vi "Data Acquisition.vi"() -> ()   [LabVIEW 2009]
panel:
  in  "Thresholding Cluster":T1={"F_DEx"=35, "F_AA"=35, " No of Bins"=100}
  out "output cluster":T2
  out "Histogram":dbl[][](graph) caption="Intensity Graph"
  in  "Current Configuration":i32
  in  "Configurations":T3(array[cluster])=[{"Configuration File Path"=path "", "Current Configuration"=TRUE}]
  in  "Time Bin (ms)":dbl=1.0 format="%.2f"
  out "APD Chart":i32[][](graph)=[[10, 21, 11, 14]]
  out "Current File Path":path
  out "Files Left To Acquire":i32
  in  "Data File I/O Information":T4={"Name of Configuration"="", "Path"=path "D:/User/Geraint/10_03_04", "File Name"="T1B18_GCW180_RAlt30um_20um_25mins_20pm_OpenAperture", "Files To Acquire"=1, "Current File Number"=3, "Time Limit"=1500.0, "Save Data"=TRUE, "Additional Comments"=""}
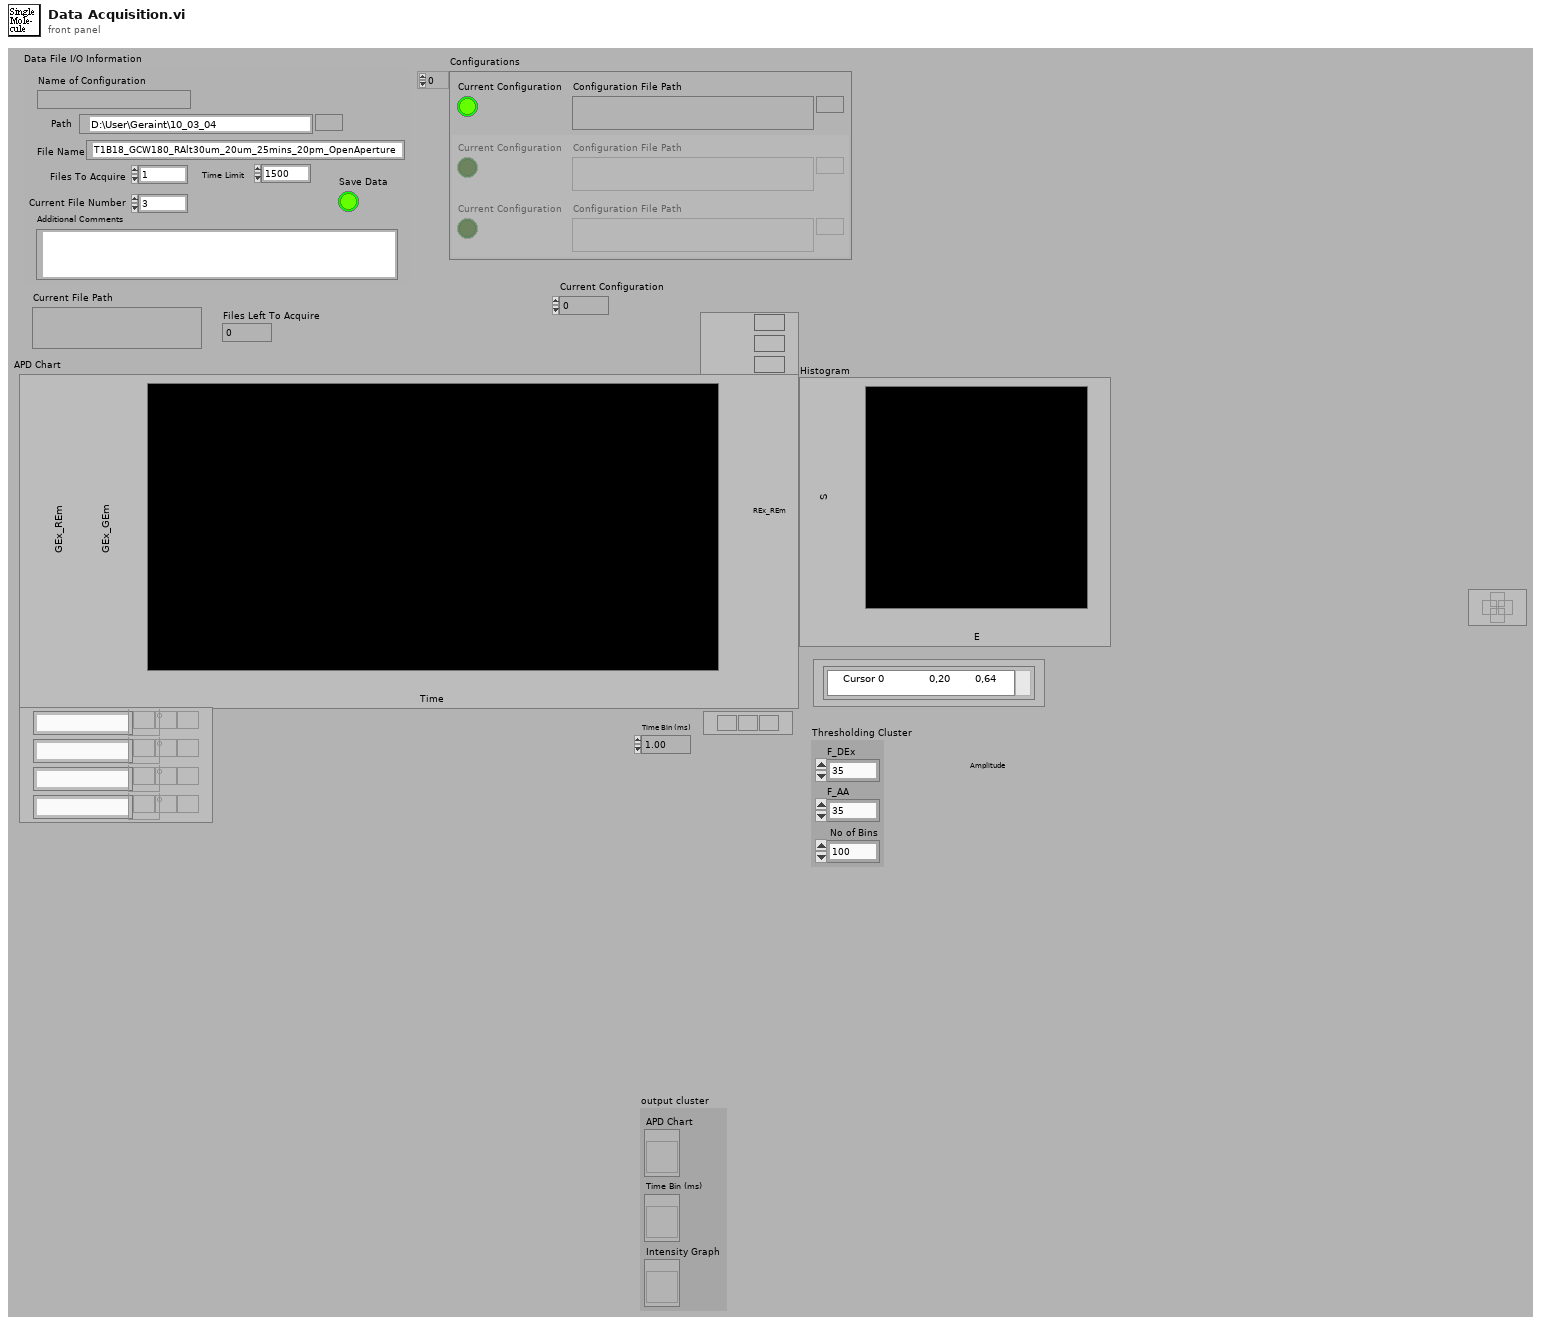
[diagram p1: front panel]
types:
  T1 = cluster{"F_DEx":i32, "F_AA":i32, " No of Bins":i32}
  T2 = cluster{"APD Chart":refnum<vi>, "Time Bin (ms)":refnum<vi>, "Intensity Graph":refnum<vi>}
  T3 = cluster{"Configuration File Path":path, "Current Configuration":bool}[]
  T4 = cluster{"Name of Configuration":string, "Path":path, "File Name":string, "Files To Acquire":i32, "Current File Number":i32, "Time Limit":dbl, "Save Data":bool, "Additional Comments":string}
  T5 = cluster{"Configuration File Path":path, "Current Configuration":bool}
  T6 = cluster{"APD Chart":refnum<vi>, "Time Bin (ms)":refnum<vi>, "Histogram":refnum<vi>}
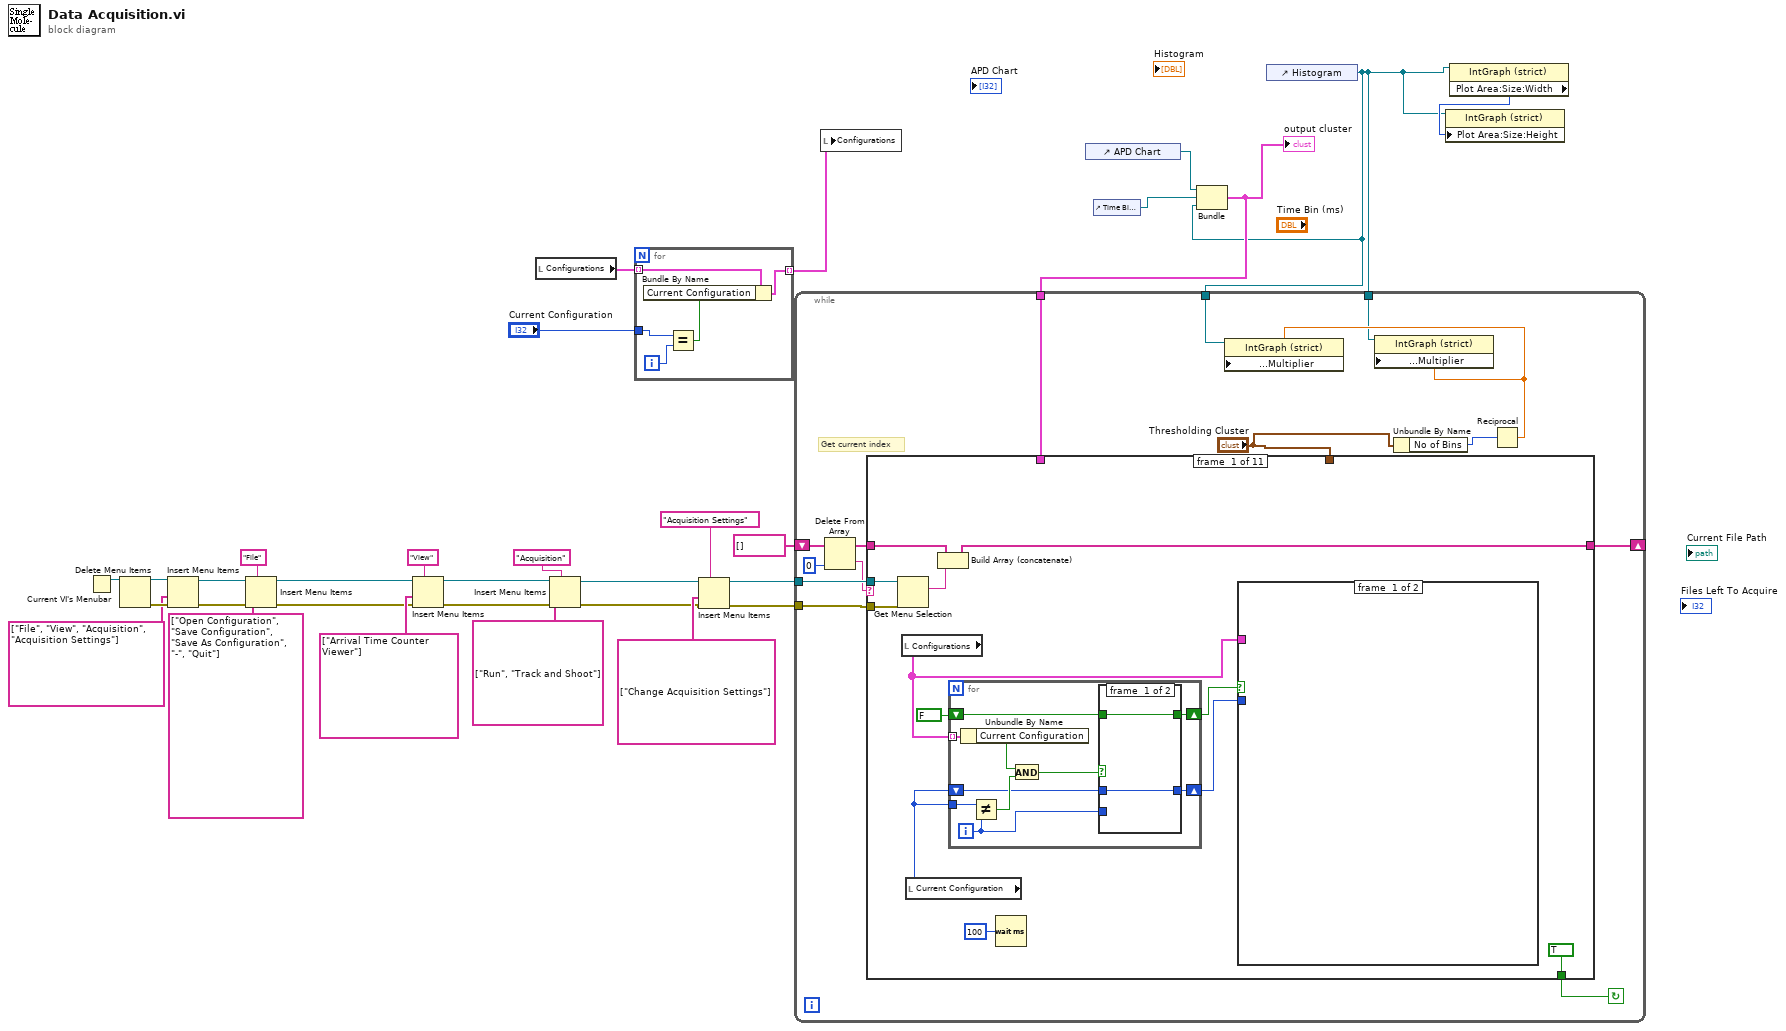
[diagram p0: block diagram]
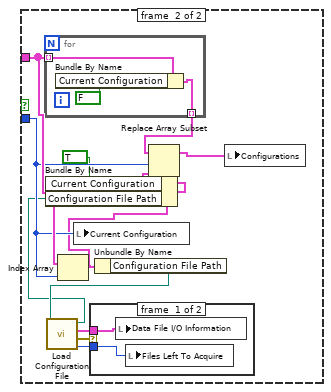
[diagram p2: hidden frame]
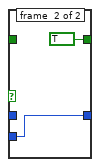
[diagram p4: hidden frame]
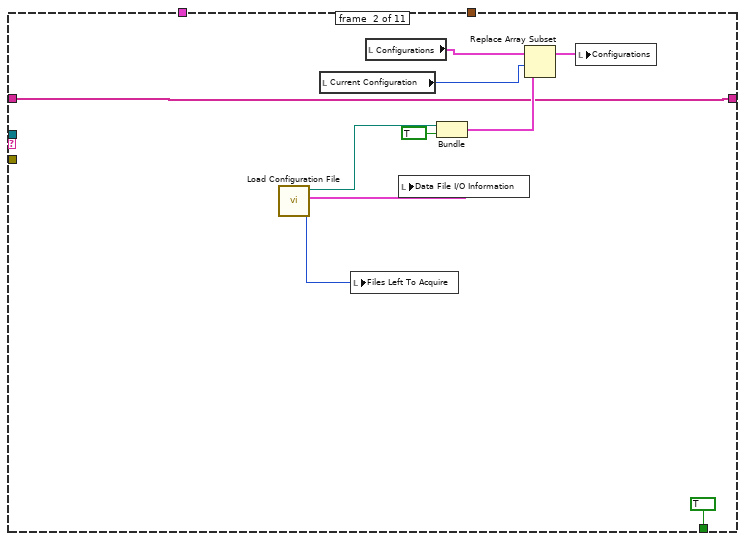
[diagram p5: hidden frame]
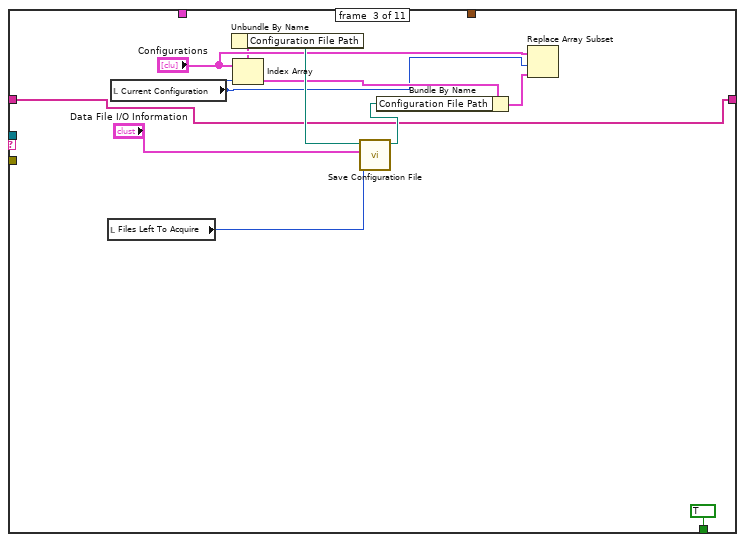
[diagram p6: hidden frame]
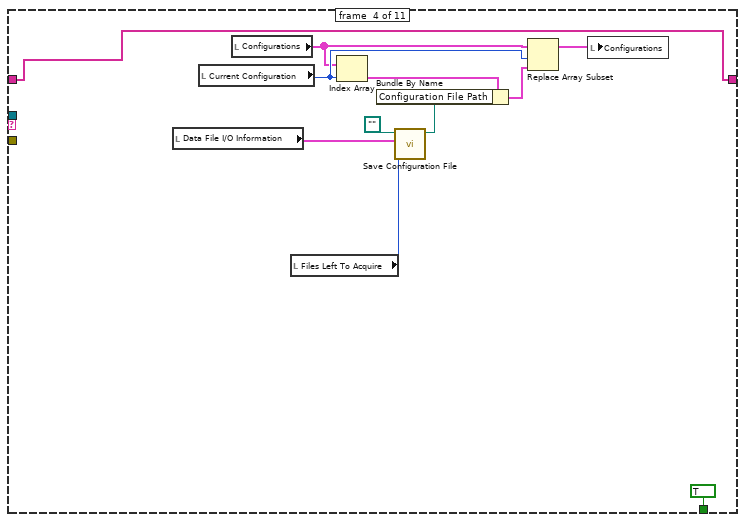
[diagram p7: hidden frame]
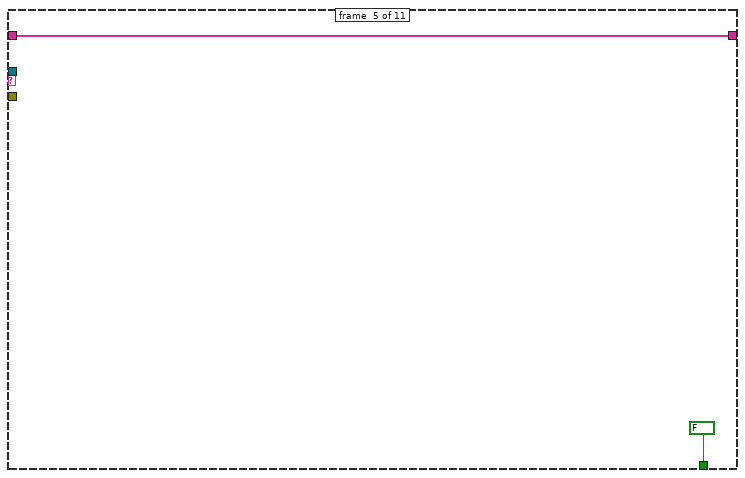
[diagram p8: hidden frame]
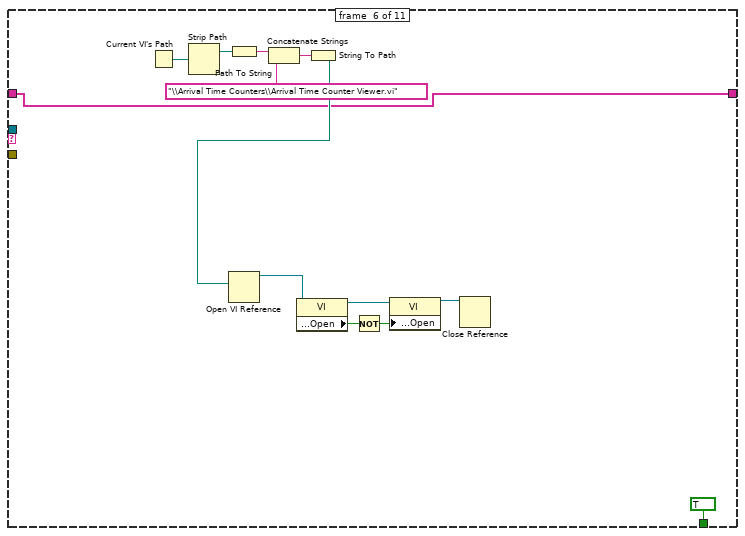
[diagram p9: hidden frame]
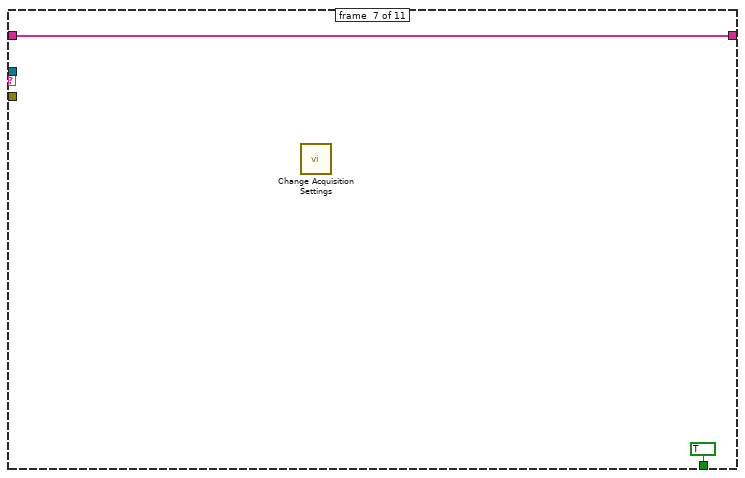
[diagram p10: hidden frame]
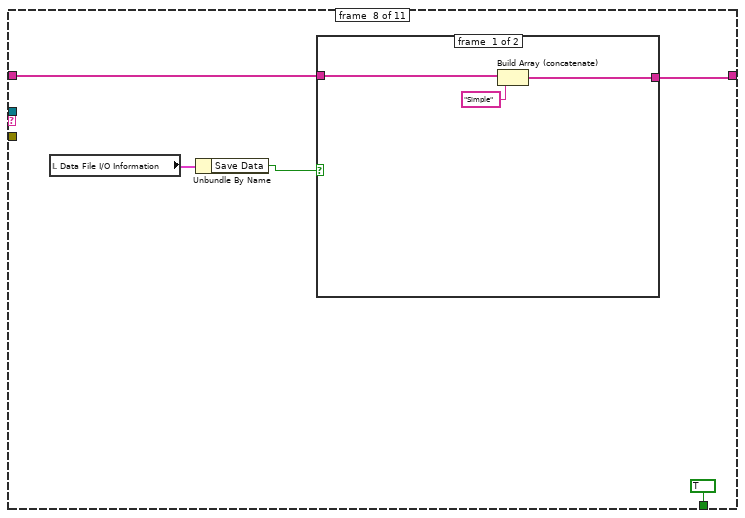
[diagram p11: hidden frame]
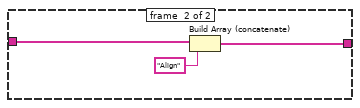
[diagram p12: hidden frame]
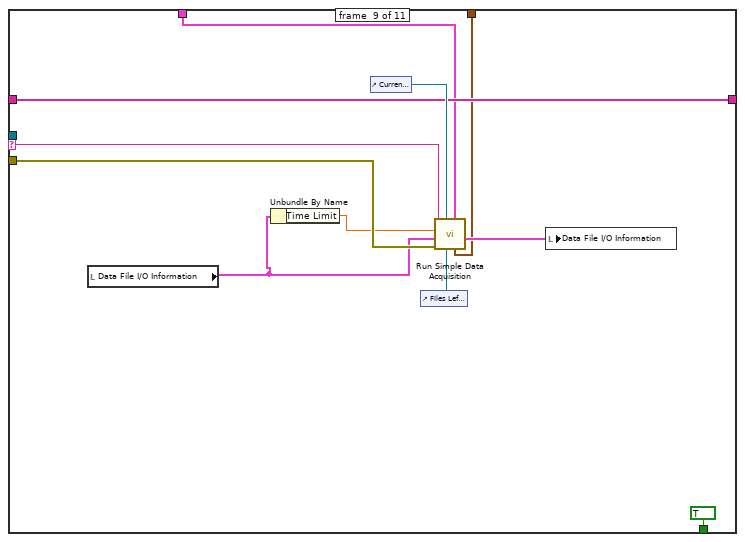
[diagram p13: hidden frame]
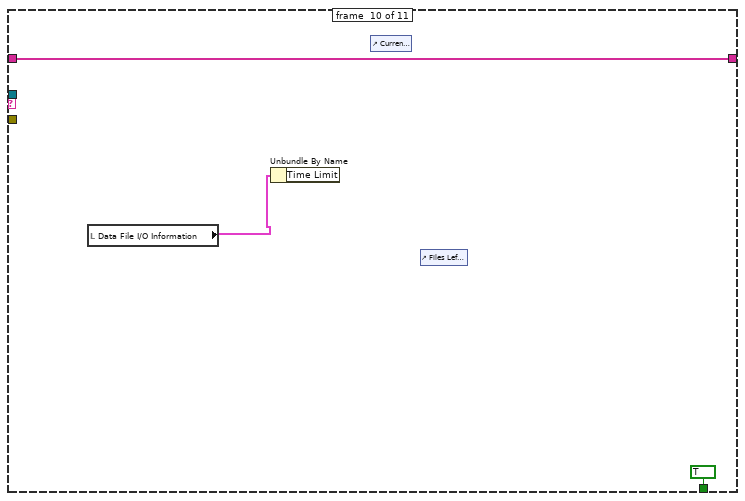
[diagram p14: hidden frame]
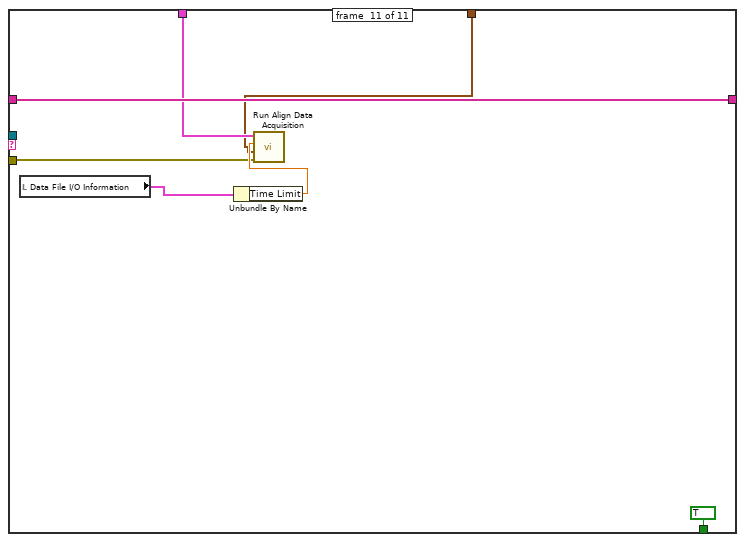
[diagram p15: hidden frame]
diagram:
  n1 = Current VI's Menubar() -> (w31:refnum<k9>)
  n2 = Delete Menu Items(9:w31) -> (0:w26:errorcluster, 3:w27:refnum<k9>)  [unwired: 3 in]
  n3 = Insert Menu Items(6:w26, 7:string[] ["File", "View", "Acquisition", "Acquisition Settings"] ("item tags"), 9:w27) -> (0:w25:errorcluster, 3:w28:refnum<k9>)  [unwired: 3 in, 1 out]
  n4 = Insert Menu Items(5:"File" ("menu tag"), 6:w25, 7:string[] ["Open Configuration", "Save Configuration", "Save As Configuration", "-", "Quit"] ("item tags"), 9:w28) -> (0:w16:errorcluster, 3:w17:refnum<k9>)  [unwired: 2 in, 1 out]
  n5 = Insert Menu Items(5:"View" ("menu tag"), 6:w16, 7:string[] ["Arrival Time Counter Viewer"] ("item tags"), 9:w17) -> (0:w15:errorcluster, 3:w14:refnum<k9>)  [unwired: 2 in, 1 out]
  n6 = local read "Configurations"() -> (w8:T3)
  n7 = Insert Menu Items(5:"Acquisition" ("menu tag"), 6:w15, 7:string[] ["Run", "Track and Shoot"] ("item tags"), 9:w14) -> (0:w12:errorcluster, 3:w13:refnum<k9>)  [unwired: 2 in, 1 out]
  n8 = for {
    tunnel: w8 -> [w36] mode=indexing
    tunnel: "Current Configuration" -> [w35]
    tunnel: [w32] -> w6 mode=indexing
    i -> [w34]
    n9 = Equal?(x=w35, y=w34) -> (x = y?=w33:bool)
    n10 = Bundle By Name(cluster=w36, "Current Configuration"=w33) -> (w32:T5)
  }
  n11 = Insert Menu Items(5:"Acquisition Settings" ("menu tag"), 6:w12, 7:string[] ["Change Acquisition Settings"] ("item tags"), 9:w13) -> (0:w10:errorcluster, 3:w11:refnum<k9>)  [unwired: 2 in, 1 out]
  n12 = local write "Configurations"(w6) -> ()
  n13 = control-ref of="APD Chart"() -> (w3:refnum<vi>)
  n14 = control-ref of="Time Bin (ms)"() -> (w9:refnum<vi>)
  n15 = control-ref of="Histogram"() -> (w1:refnum<vi>)
  n16 = Bundle("APD Chart"=w3, "Time Bin (ms)"=w9, "Histogram"=w1) -> (w4:T6)  [unwired: 1 in]
  "output cluster" <- w4
  n17 = while {
    tunnel: w10 -> [w47]
    tunnel: w11 -> [w48]
    tunnel: w4 -> [w49]
    shift-right: [w46] -> _
    shift-left: string[] [] -> [w44]
    tunnel: w1 -> [w38]
    tunnel: w1 -> [w37]
    stop <- w50 continue-if-true
    # "Get current index"
    n18 = Delete From Array(array=w44, index=0) -> (deleted portion=w42:string, array with subset deleted=w45:string[])  [unwired: 1 in]
    n19 = case shown="\"Save Configuration\"" w42 {
      selector: w42 -> [_ _ _ _ _ _ _ _ w161 _ _]
      tunnel: [TRUE TRUE TRUE TRUE FALSE TRUE TRUE TRUE TRUE TRUE TRUE] -> w50
      tunnel: w47 -> [w54 _ _ _ _ _ _ _ w163 _ w169]
      tunnel: w49 -> [_ _ _ _ _ _ _ _ w154 _ w168]
      tunnel: w48 -> [w55 _ _ _ _ _ _ _ _ _ _]
      tunnel: [w52 w94 w105 w114 w125 w127 w140 w143 w157 w165 w172] -> w46
      tunnel: w45 -> [w51 w94 w105 w114 w125 w127 w140 w144 w157 w165 w172]
      tunnel: "Thresholding Cluster" -> [_ _ _ _ _ _ _ _ w153 _ w167]
      frame #0 {
        n20 = Get Menu Selection(0:w55, 3:w54) -> (6:w53:string)  [unwired: 2 in, 4 out]
        n21 = local read "Configurations"() -> (w60:T3)
        n22 = local read "Current Configuration"() -> (w57:i32)
        n23 = Build Array (concatenate)(w51, w53) -> (w52:string[])
        n24 = for {
          tunnel: w60 -> [w89] mode=indexing
          shift-right: [w85] -> w59
          shift-left: w57 -> [w86]
          shift-right: [w81] -> w58
          shift-left: FALSE -> [w82]
          tunnel: w57 -> [w80]
          i -> [w84]
          n25 = Unbundle By Name(w89) -> ("Current Configuration"=w88:bool)
          n26 = Not Equal?(x=w80, y=w84) -> (x != y?=w87:bool)
          n27 = And(x=w88, y=w87) -> (x .and. y?=w83:bool)
          n28 = case shown="True" w83 {
            tunnel: w86 -> [w91 _]
            tunnel: [w91 w93] -> w85
            tunnel: w84 -> [_ w93]
            tunnel: w82 -> [w90 _]
            tunnel: [w90 TRUE] -> w81
            frame #0 {
            }
            frame #1 {
            }
          }
        }
        n29 = Wait (ms)(milliseconds to wait=u32 100) -> ()  [unwired: 1 out]
        n30 = case shown="True" w58 {
          tunnel: w60 -> [_ w70]
          tunnel: w59 -> [_ w67]
          frame #0 {
          }
          frame #1 {
            n31 = for {
              tunnel: w70 -> [w79] mode=indexing
              tunnel: [w78] -> w69 mode=indexing
              n32 = Bundle By Name(cluster=w79, "Current Configuration"=FALSE) -> (w78:T5)
            }
            n33 = Index Array(array=w70, index=w67) -> (element=w66:T5)
            n34 = local write "Current Configuration"(w67) -> ()
            n35 = Unbundle By Name(w66) -> ("Configuration File Path"=w74:path)
            n36 = call "Load Configuration File.vi"("New File Path"=w74) -> ("Files To Acquire"=w72:i32, "error"=w71:errorcluster, "Data File I/O Information"=w73:T4, "new file path"=w64:path)  [unwired: 7 in]
            n37 = Bundle By Name(cluster=w66, "Current Configuration"=TRUE, "Configuration File Path"=w64) -> (w65:T5)
            n38 = case shown="No Error" w71 {
              tunnel: w73 -> [w76 _]
              tunnel: w72 -> [w75 _]
              frame #0 {
                n39 = local write "Data File I/O Information"(w76) -> ()
                n40 = local write "Files Left To Acquire"(w75) -> ()
              }
              frame #1 {
              }
            }
            n41 = Replace Array Subset(array=w69, new element=w65, index=w67) -> (w68:T3)
            n42 = local write "Configurations"(w68) -> ()
          }
        }
      }
      frame #1 {
        n43 = call "Load Configuration File.vi"() -> ("Files To Acquire"=w101:i32, "Data File I/O Information"=w102:T4, "new file path"=w100:path)  [unwired: 8 in, 1 out]
        n44 = local read "Current Configuration"() -> (w97:i32)
        n45 = local write "Files Left To Acquire"(w101) -> ()
        n46 = local read "Configurations"() -> (w98:T3)
        n47 = local write "Data File I/O Information"(w102) -> ()
        n48 = Bundle("new file path"=w100, TRUE) -> (w96:cluster{"new file path":path, bool})  [unwired: 1 in]
        n49 = Replace Array Subset(array=w98, new element=w96, index=w97) -> (w95:T3)
        n50 = local write "Configurations"(w95) -> ()
      }
      frame #2 {
        n51 = local read "Files Left To Acquire"() -> (w112:i32)
        n52 = local read "Current Configuration"() -> (w106:i32)
        n53 = Index Array(array="Configurations", index=w106) -> (element=w107:T5)
        n54 = Unbundle By Name(w107) -> ("Configuration File Path"=w111:path)
        n55 = call "Save Configuration File.vi"("Files To Acquire"=w112, "Data File I/O Information"="Data File I/O Information", "Configuration File Path"=w111) -> ("new file path"=w108:path)  [unwired: 8 in]
        n56 = Bundle By Name(cluster=w107, "Configuration File Path"=w108) -> (w110:T5)
        n57 = Replace Array Subset(array="Configurations", new element=w110, index=w106) -> ()  [unwired: 1 out]
      }
      frame #3 {
        n58 = local read "Data File I/O Information"() -> (w123:T4)
        n59 = local read "Current Configuration"() -> (w117:i32)
        n60 = local read "Configurations"() -> (w116:T3)
        n61 = local read "Files Left To Acquire"() -> (w121:i32)
        n62 = Index Array(array=w116, index=w117) -> (element=w120:T5)
        n63 = call "Save Configuration File.vi"("Files To Acquire"=w121, "Data File I/O Information"=w123, "Configuration File Path"=path "") -> ("new file path"=w119:path)  [unwired: 8 in]
        n64 = Bundle By Name(cluster=w120, "Configuration File Path"=w119) -> (w118:T5)
        n65 = Replace Array Subset(array=w116, new element=w118, index=w117) -> (w115:T3)
        n66 = local write "Configurations"(w115) -> ()
      }
      frame #4 {
      }
      frame #5 {
        n67 = Current VI's Path() -> (path=w133:path)
        n68 = Strip Path(path=w133) -> (stripped path=w132:path)  [unwired: 1 out]
        n69 = Path To String(path=w132) -> (string=w131:string)
        n70 = Concatenate Strings(w131, "\\Arrival Time Counters\\Arrival Time Counter Viewer.vi") -> (w129:string)
        n71 = String To Path(string=w129) -> (path=w128:path)
        n72 = Open VI Reference(vi path=w128) -> (vi reference=w138:refnum<vi>)  [unwired: 5 in, 1 out]
        n73 = property class="VI"(reference=w138) -> (reference out=w137:refnum<vi>, "Front Panel Window:Open"=w136:bool)  [unwired: 1 in, 1 out]
        n74 = Not(x=w136) -> (.not. x?=w135:bool)
        n75 = property class="VI"(reference=w137, "Front Panel Window:Open"=w135) -> (reference out=w134:refnum<vi>)  [unwired: 1 in, 1 out]
        n76 = Close Reference(reference=w134) -> ()  [unwired: 1 in, 1 out]
      }
      frame #6 {
        n77 = call "Change Acquisition Settings.vi"() -> ()  [unwired: 1 in]
      }
      frame #7 {
        n78 = local read "Data File I/O Information"() -> (w146:T4)
        n79 = Unbundle By Name(w146) -> ("Save Data"=w145:bool)
        n80 = case shown="False" w145 {
          tunnel: w144 -> [w149 w152]
          tunnel: [w147 w150] -> w143
          frame #0 {
            n81 = Build Array (concatenate)(w149, "Simple") -> (w147:string[])
          }
          frame #1 {
            n82 = Build Array (concatenate)(w152, "Align") -> (w150:string[])
          }
        }
      }
      frame #8 {
        n83 = local read "Data File I/O Information"() -> (w156:T4)
        n84 = Unbundle By Name(w156) -> ("Time Limit"=w155:dbl)
        n85 = control-ref of="Current File Path"() -> (w159:refnum<vi>)
        n86 = control-ref of="Files Left To Acquire"() -> (w158:refnum<vi>)
        n87 = call "Run Simple Data Acquisition.vi"("Thresholding Cluster"=w153, "output cluster 2"=w154, "Files To Acquire Refnum"=w158, "Path Refnum"=w159, "error in"=w163, "Data File I/O Information"=w156, "Time Limit"=w155, "File Type"=w161) -> ("Data File I/O Information"=w160:T4)  [unwired: 2 in, 1 out]
        n88 = local write "Data File I/O Information"(w160) -> ()
      }
      frame #9 {
        n89 = local read "Data File I/O Information"() -> (w164:T4)
        n90 = Unbundle By Name(w164) -> ()  [unwired: 1 out]
        n91 = control-ref of="Current File Path"() -> ()  [unwired: 1 out]
        n92 = control-ref of="Files Left To Acquire"() -> ()  [unwired: 1 out]
      }
      frame #10 {
        n93 = local read "Data File I/O Information"() -> (w171:T4)
        n94 = Unbundle By Name(w171) -> ("Time Limit"=w170:dbl)
        n95 = call "Run Align Data Acquisition.vi"("error in"=w169, "Thresholding Cluster 2"=w167, "Time Limit"=w170, "output cluster 2"=w168) -> ()  [unwired: 7 in, 1 out]
      }
    }
    n96 = Unbundle By Name("Thresholding Cluster") -> ("No of Bins"=w40:i32)
    n97 = Reciprocal(x=w40) -> (1/x=w41:dbl)
    n98 = property class="IntGraph (strict)"(reference=w37, "Y Scale.Offset and Multiplier:Multiplier"=w41) -> ()  [unwired: 1 in, 2 out]
    n99 = property class="IntGraph (strict)"(reference=w38, "X Scale.Offset and Multiplier:Multiplier"=w41) -> ()  [unwired: 1 in, 2 out]
  }
  n100 = property class="IntGraph (strict)"(reference=w1) -> ("Plot Area:Size:Width"=w2:u32)  [unwired: 1 in, 2 out]
  n101 = property class="IntGraph (strict)"(reference=w1, "Plot Area:Size:Height"=w2) -> ()  [unwired: 1 in, 2 out]
